vi "Initialize.vi"(8 "error in (no error)":errorcluster, 11 "test handler in":refnum<class "Test Handler.lvclass">) -> (0 "error out":errorcluster, 3 "test handler out":refnum<class "Test Handler.lvclass">)   [LabVIEW 2018, in "Test Handler.lvclass"]
uses:
  Test Handler.lvclass
  Test Handler.lvclass/Test Handler.ctl
  src/api/extension/formatting_handler_interface/Formatting Handler.lvclass
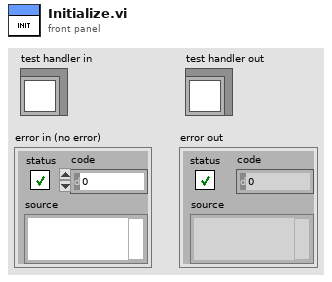
[diagram p1: front panel]
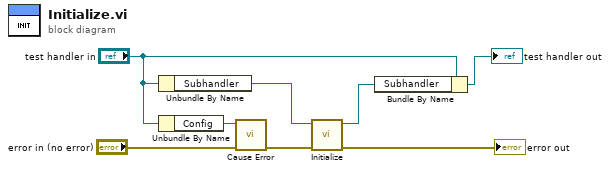
[diagram p0: block diagram]
diagram:
  n1 = Unbundle By Name("test handler in") -> ("Subhandler"=w5:refnum<class "Formatting Handler.lvclass">)
  n2 = Unbundle By Name("test handler in") -> ("Config"=w7:path)
  n3 = call "Cause Error.vi"("error in (no error)"="error in (no error)", "ini file path"=w7) -> ("error out"=w2:errorcluster)  [unwired: 8 in, 1 out]
  n4 = call-dynamic "Initialize.vi"("error in (no error)"=w2, "handler in"=w5) -> ("error out"=→"error out":errorcluster, "handler out"=w3:refnum<class "Formatting Handler.lvclass">)  [unwired: 8 in]
  n5 = Bundle By Name(cluster="test handler in", "Subhandler"=w3) -> (→"test handler out":refnum<class "Test Handler.lvclass">)
